vi "Main.vi"(8 "error in":errorcluster, 11 "Message Log in":refnum<class "Message Log.lvclass">) -> (0 "error out":errorcluster, 3 "Message Log out":refnum<class "Message Log.lvclass">)   [LabVIEW 2017, in "Message Log.lvclass"]
doc: "The <b>Queued Message Handler</b> of the Worker that owns this VI."
uses:
  Message Log.lvclass
  C:/Program Files (x86)/National Instruments/LabVIEW 2017/vi.lib/addons/_Workers/Library/Classes/Worker/Worker.lvclass
  Message Log Columns.ctl
  Buttons/Sort Button.ctl
  Buttons/Logging Button.ctl
  Buttons/Clear Filter Button.ctl
  Buttons/Undo Filter Button.ctl
  Buttons/Filter Button.ctl
  Buttons/Resize Button.ctl
  Buttons/Pause Button.ctl
  Buttons/WID Button.ctl
  Buttons/Open Application Manager.ctl
  <vilib>/Utility/miscctls.llb/LVRowAndColumnUnsignedTypeDef.ctl
  FP Refs.ctl
  Message Log.lvclass/Message Log.ctl
  <vilib>/addons/_Workers/Library/Classes/Worker/Worker.lvclass/Worker.ctl
  rql_Update Message Log Columns.ctl
  rql_EHL Logging - Value Change.ctl
  rql_EHL Pause - Value Change.ctl
  rql_EHL WID - Value Change.ctl
  Initialization Data.ctl
  Response Cases.ctl
  <vilib>/addons/_Workers/Library/Case Label.ctl
  Common VIs/Message Log ID.ctl
  Config Data.ctl
  <vilib>/Utility/miscctls.llb/LVRectTypeDef.ctl
  <vilib>/addons/_Workers/Library/Classes/Message/Priority.ctl
  rsp_Message Log Shutdown.ctl
  rsp_Message Log Exited.ctl
  Message Log Filter Data.ctl
  String Filter Type.ctl
  rql_EHL Message Log - Mouse Down.ctl
  Listbox Selection.ctl
  <vilib>/Utility/miscctls.llb/LVRowAndColumnTypeDef.ctl
  rql_EHL Sort - Value Change.ctl
  rql_EHL Resize - Value Change.ctl
  rql_EHL Undo Filter - Value Change.ctl
  rqp_Show Front Panel.ctl
  rwr_Get Shutdown Data Reply.ctl
  rqp_Filter as Enque Worker.ctl
  rqp_Filter as Deque Worker.ctl
  Format Message Log Data.vi
  Log Message to File.vi
  Replace ID with Alias.vi
  <vilib>/Platform/browser.llb/Open URL in Default Browser (string).vi
  <vilib>/addons/_Workers/Library/Classes/Worker/Worker.lvclass
  <vilib>/addons/_Workers/Library/Workers.lvlib
  <vilib>/addons/_Workers/Library/Classes/Message Queue/Message Queue.lvclass
  <vilib>/addons/_Workers/Library/Classes/Message/Message.lvclass
panel:
  in  "Show App Mgr":T1
  out "Warning : Message Backlog":i32
  out "Visible ML Columns":bool[](array[boolean])
  out "Title":string="Worker A  (127.0.0.1)"
  in  "WID":T2
  in  "Pause":T3
  in  "Resize":T4
  in  "Filter":T5
  in  "Undo":T6
  in  "Clear":T7
  in  "Logging":T8
  in  "Filter String":string caption="String to Filter"
  in  "Sort":T9
  in  "Column":T10
  in  "Filter Type":enum16{"string only", "match pattern"}(ring)
  in  "Filter Log":i32(listbox)=-1
  in  "Message Log":i32(listbox)=-1
  out "Message Box":string
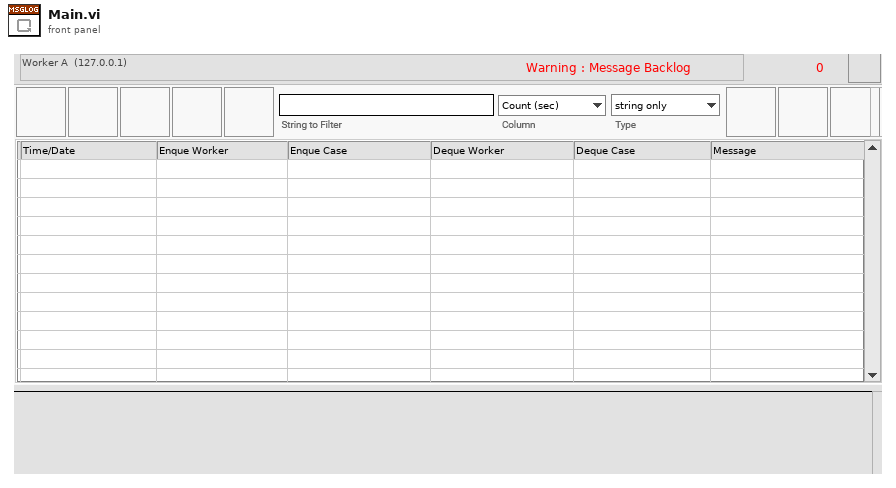
[diagram p1: front panel]
types:
  T1 = typedef "Open Application Manager.ctl" = bool
  T2 = typedef "WID Button.ctl" = bool
  T3 = typedef "Pause Button.ctl" = bool
  T4 = typedef "Resize Button.ctl" = bool
  T5 = typedef "Filter Button.ctl" = bool
  T6 = typedef "Undo Filter Button.ctl" = bool
  T7 = typedef "Clear Filter Button.ctl" = bool
  T8 = typedef "Logging Button.ctl" = bool
  T9 = typedef "Sort Button.ctl" = bool
  T10 = typedef "Message Log.lvclass/Message Log Columns.ctl" = enum16{"Count (sec)", "Time/Date", "Enque Worker", "Enque Case", "Deque Worker", "Deque Case", "Priority", "Message"}
  T11 = typedef "Message Log.lvclass/FP Refs.ctl" = cluster{"Message Log.Ref":refnum<vi>, "VisibleMLColumns.Ref":refnum<vi>, "Filter Type.Ref":refnum<vi>, "Column.Ref":refnum<vi>, "Filter String.Ref":refnum<vi>, "Filter Log.Ref":refnum<vi>, "MessageBox.Ref":refnum<vi>, "MessageBacklog.Ref":refnum<vi>, "Title.Ref":refnum<vi>}
  T12 = typedef "LVRowAndColumnUnsignedTypeDef.ctl" = cluster{"Row":u32, "Column":u32}
  T13 = typedef "LVPointTypeDef.ctl" = cluster{"Horizontal":i16, "Vertical":i16}
  T14 = typedef "Message Log.lvclass/Initialization Data.ctl" = cluster{"Response Cases":T15, "Message Log ID":T17, "Config Data":T18}
  T15 = typedef "Message Log.lvclass/Response Cases.ctl" = cluster{"Message Log Exited":T16, "Go to MHL Case":T16, "Open Running VI":T16, "Message Log Shutdown Data":T16, "Show Application Manager":T16}
  T16 = typedef "Workers.lvlib/Case Label.ctl" = string
  T17 = typedef "Message Log ID.ctl" = cluster{"Head Worker ID":string, "IP Address":string}
  T18 = typedef "Message Log.lvclass/Config Data.ctl" = cluster{"Max Num Rows":i32, "Visible Columns":bool[], "Splitter Position":i32, "Column Widths":u32[], "WinBounds":T19, "FP.State":enum32{"Invalid", "Standard", "Closed", "Hidden", "Minimized", "Maximized"}, "Monitor":u16, "Logging":bool, "LogBaseFolder":path}
  T19 = typedef "LVRectTypeDef.ctl" = cluster{"Left":i16, "Top":i16, "Right":i16, "Bottom":i16}
  T20 = typedef "Workers.lvlib/Message.lvclass/Priority.ctl" = enum16{"Low", "Normal", "High"}
  T21 = typedef "Message Log.lvclass/rql_Update Message Log Columns.ctl" = cluster{"Boolean":bool}
  T22 = typedef "Message Log.lvclass/rsp_Message Log Shutdown.ctl" = cluster{"Config Data":T18}
  T23 = typedef "Message Log.lvclass/rsp_Message Log Exited.ctl" = cluster{"Message Log ID":T17}
  T24 = typedef "Message Log.lvclass/Message Log Filter Data.ctl" = cluster{"Element":string, "Column":T10, "Filter Type":T25}
  T25 = typedef "Message Log.lvclass/String Filter Type.ctl" = enum16{"string only", "match pattern"}
  T26 = typedef "Message Log.lvclass/rql_EHL Message Log - Mouse Down.ctl" = cluster{"Listbox Selection":T27}
  T27 = typedef "Message Log.lvclass/Listbox Selection.ctl" = cluster{"Cell Position":T28, "Row":string[]}
  T28 = typedef "LVRowAndColumnTypeDef.ctl" = cluster{"Row":i32, "Column":i32}
  T29 = typedef "Message Log.lvclass/rql_EHL Pause - Value Change.ctl" = cluster{"Boolean":bool}
  T30 = typedef "Message Log.lvclass/rql_EHL WID - Value Change.ctl" = cluster{"Boolean":bool}
  T31 = typedef "Message Log.lvclass/rql_EHL Sort - Value Change.ctl" = cluster{"String":string}
  T32 = typedef "Message Log.lvclass/rql_EHL Resize - Value Change.ctl" = cluster{"String":string}
  T33 = typedef "Message Log.lvclass/rql_EHL Undo Filter - Value Change.ctl" = cluster{"String":string}
  T34 = typedef "Message Log.lvclass/rql_EHL Logging - Value Change.ctl" = cluster{"Boolean":bool}
  T35 = typedef "Message Log.lvclass/rqp_Show Front Panel.ctl" = cluster{"String":string}
  T36 = typedef "Message Log.lvclass/rwr_Get Shutdown Data Reply.ctl" = cluster{"Config Data":T18}
  T37 = typedef "Message Log.lvclass/rqp_Filter as Enque Worker.ctl" = cluster{"Worker ID":string}
  T38 = typedef "Message Log.lvclass/rqp_Filter as Deque Worker.ctl" = cluster{"Worker ID":string}
  T39 = typedef "LVPoint32TypeDef.ctl" = cluster{"Horizontal":i32, "Vertical":i32}
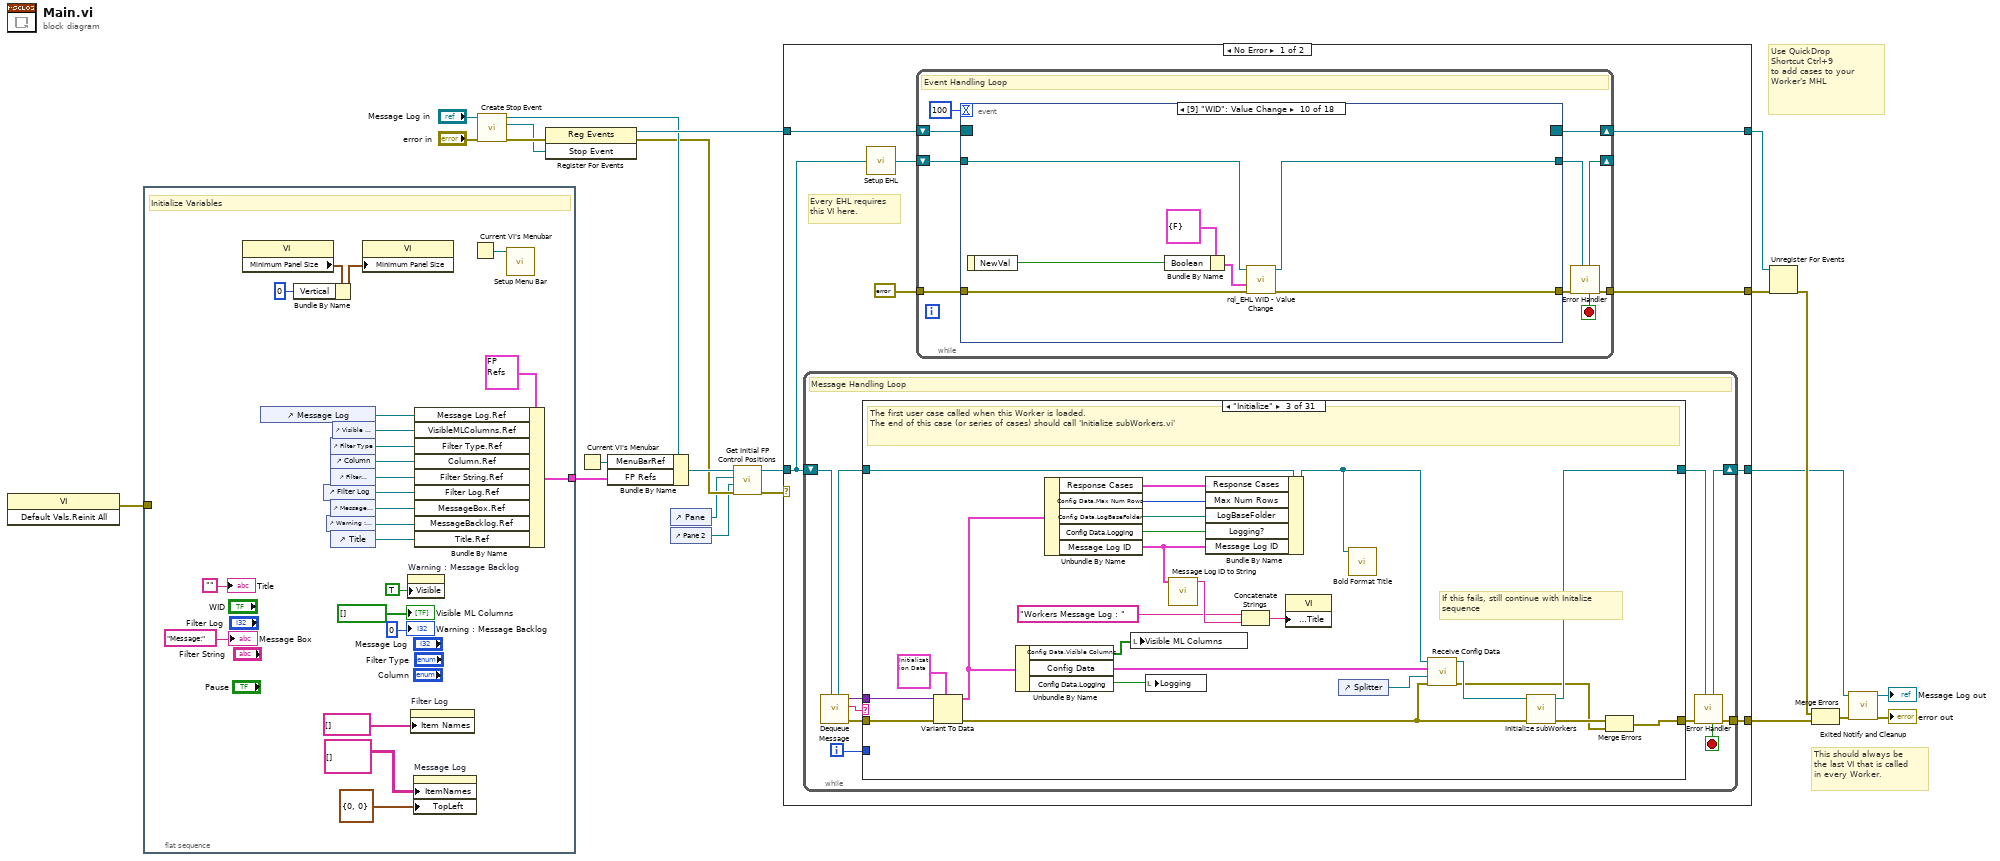
[diagram p0: block diagram]
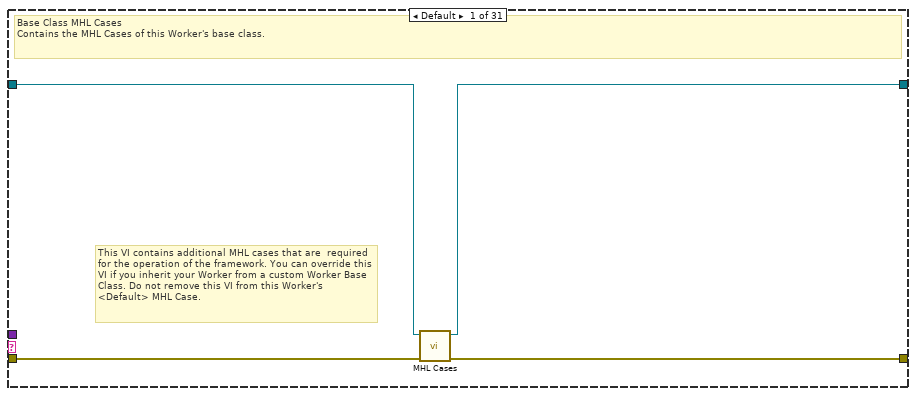
[diagram p2: hidden frame]
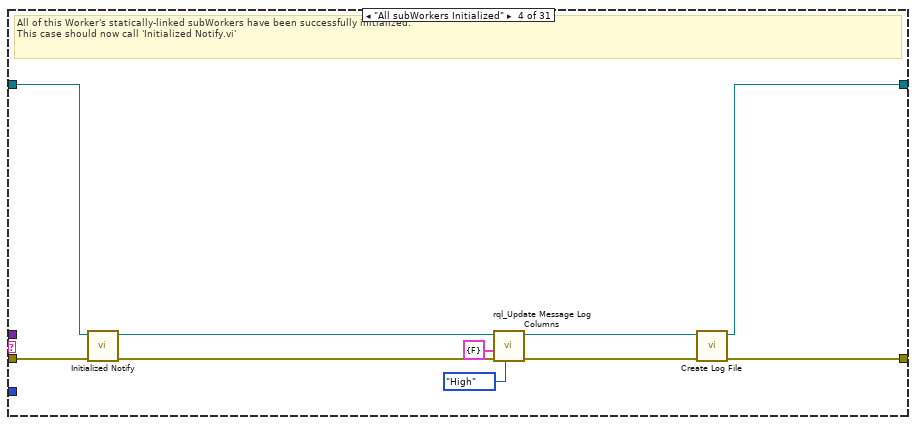
[diagram p4: hidden frame]
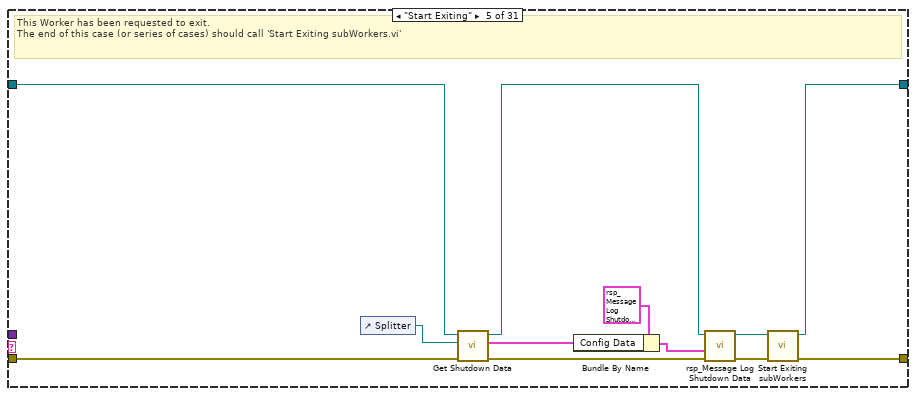
[diagram p5: hidden frame]
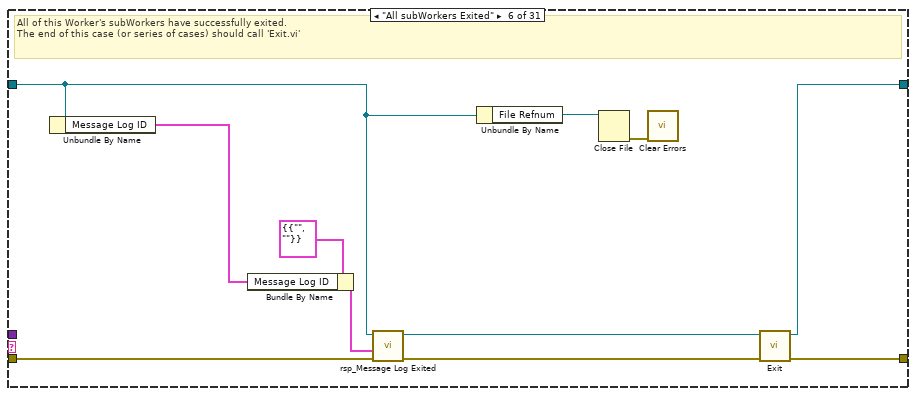
[diagram p6: hidden frame]
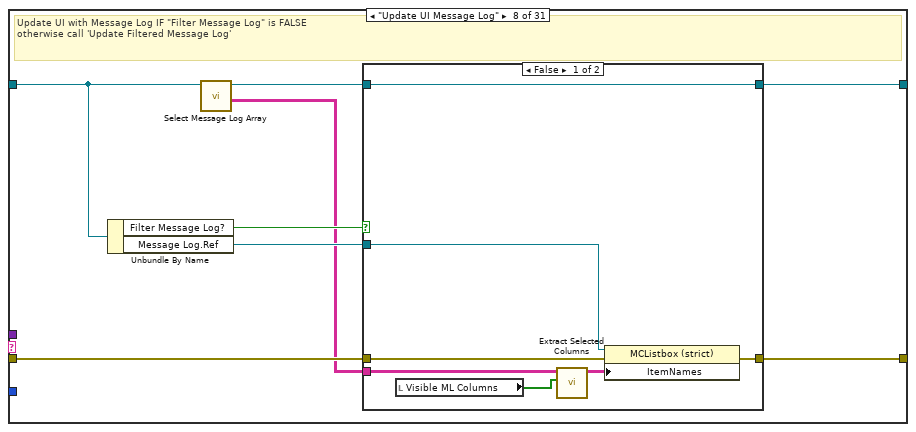
[diagram p8: hidden frame]
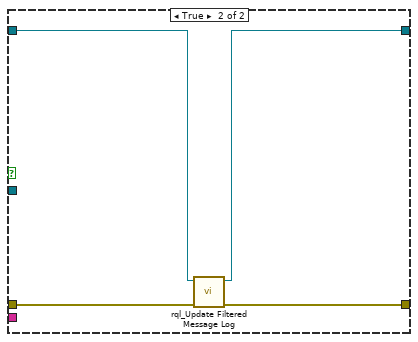
[diagram p9: hidden frame]
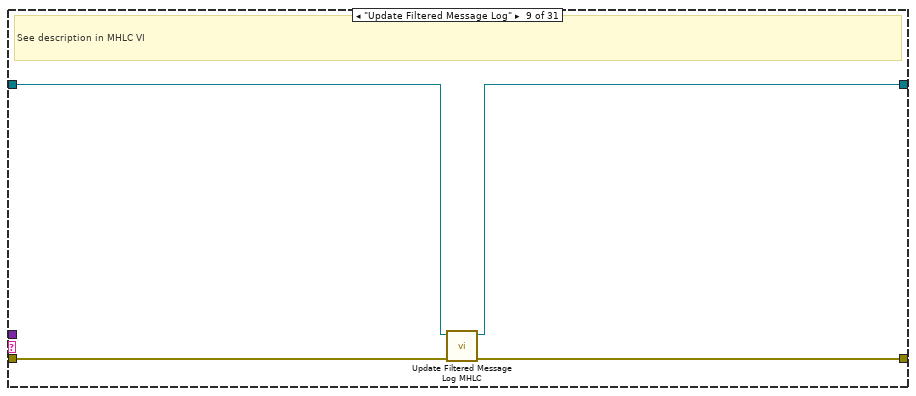
[diagram p10: hidden frame]
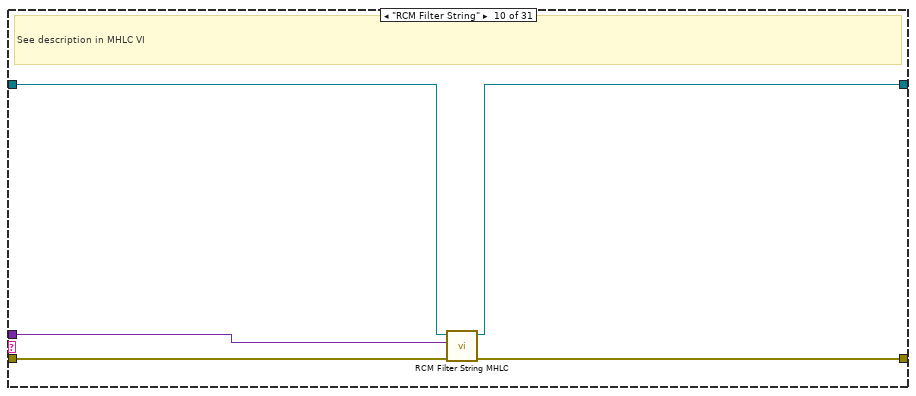
[diagram p11: hidden frame]
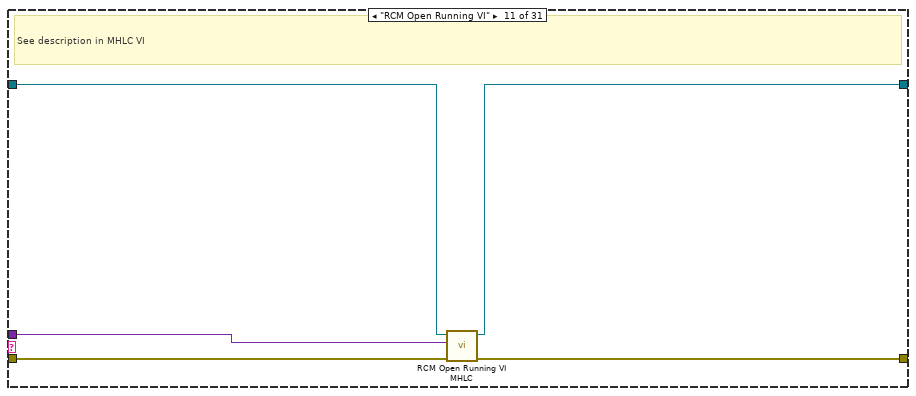
[diagram p12: hidden frame]
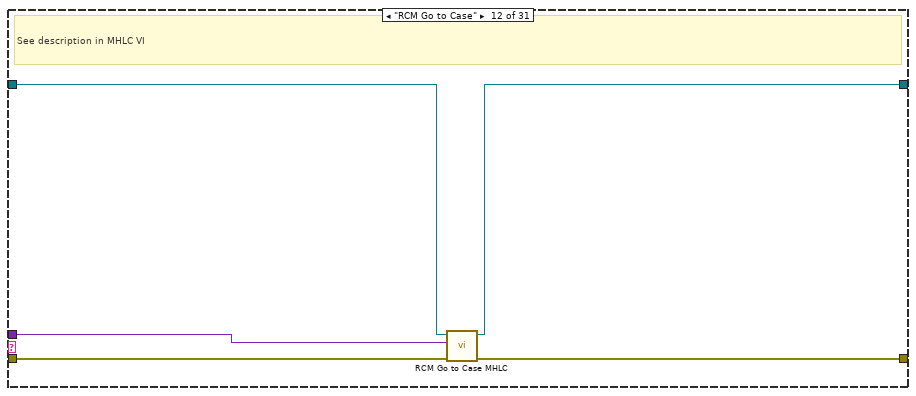
[diagram p13: hidden frame]
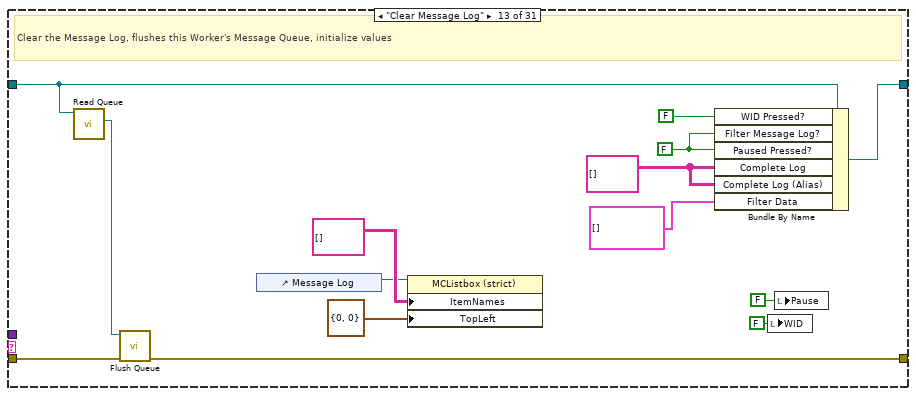
[diagram p14: hidden frame]
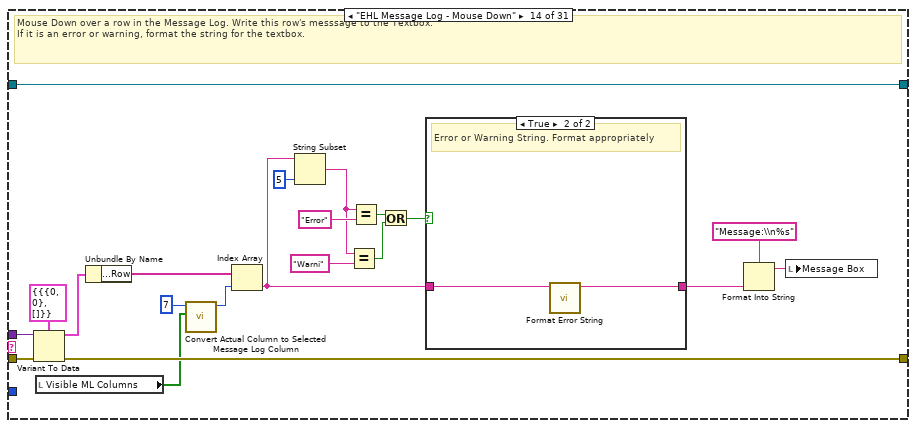
[diagram p15: hidden frame]
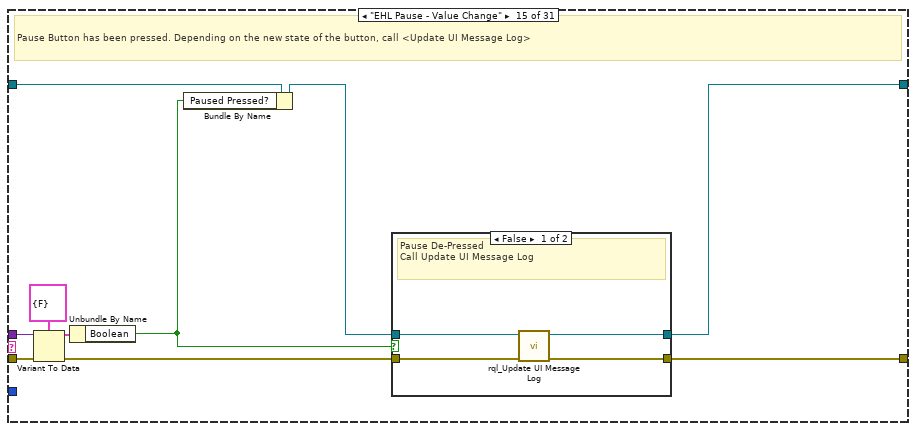
[diagram p17: hidden frame]
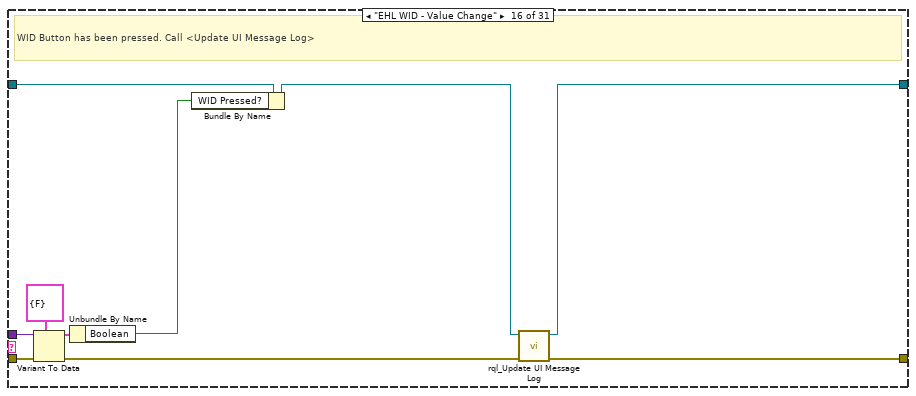
[diagram p19: hidden frame]
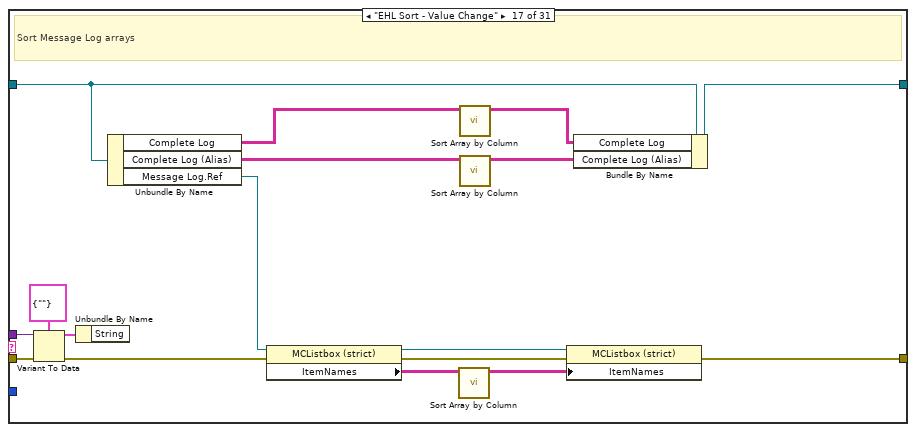
[diagram p20: hidden frame]
diagram:
  # "Use QuickDrop\nShortcut Ctrl+9\nto add cases to your\nWorker's MHL"
  # "This should always be the last VI that is called in every Worker."
  n1 = invoke class="VI" method="Default Vals.Reinit All"() -> (error out=w10:errorcluster)  [unwired: 3 in, 2 out]
  n2 = flat-sequence {
    tunnel: w10 -> [_]
    tunnel: [w45] -> w8
    frame #0 {
      # "Initialize Variables"
      n3 = property class="VI"() -> ("Minimum Panel Size"=w32:T13)  [unwired: 2 in, 2 out]
      n4 = control-ref of="Message Log"() -> (w44:refnum<vi>)
      n5 = Bundle By Name(cluster=w32, "Vertical"=i16 0) -> (w31:T13)
      n6 = control-ref of="Filter Log"() -> (w40:refnum<vi>)
      n7 = control-ref of="Warning : Message Backlog"() -> (w38:refnum<vi>)
      n8 = control-ref of="Filter Type"() -> (w42:refnum<vi>)
      n9 = control-ref of="Column"() -> (w26:refnum<vi>)
      n10 = control-ref of="Filter String"() -> (w41:refnum<vi>)
      n11 = control-ref of="Message Box"() -> (w39:refnum<vi>)
      n12 = control-ref of="Title"() -> (w25:refnum<vi>)
      n13 = control-ref of="Visible ML Columns"() -> (w43:refnum<vi>)
      n14 = property class="VI"("Minimum Panel Size"=w31) -> ()  [unwired: 2 in, 2 out]
      n15 = property on="Warning : Message Backlog" class="DigNum (strict)"("Visible"=TRUE) -> ()  [unwired: 2 in, 2 out]
      n16 = property on="Filter Log" class="LstBox (strict)"("Item Names"=string[] [] ("Sorted Array Out")) -> ()  [unwired: 2 in, 2 out]
      n17 = property on="Message Log" class="MCListbox (strict)"("ItemNames"=string[][] [] ("Sorted Array Out"), "TopLeft"=T12 {"Row"=0, "Column"=0} ("Top Left Visible Cell")) -> ()  [unwired: 2 in, 2 out]
      n18 = Bundle By Name(cluster=T11 {"Message Log.Ref"=refnum, "VisibleMLColumns.Ref"=refnum, "Filter Type.Ref"=refnum, "Column.Ref"=refnum, "Filter String.Ref"=refnum, "Filter Log.Ref"=refnum, "MessageBox.Ref"=refnum, "MessageBacklog.Ref"=refnum, "Title.Ref"=refnum} ("Data"), "Message Log.Ref"=w44, "VisibleMLColumns.Ref"=w43, "Filter Type.Ref"=w42, "Column.Ref"=w26, "Filter String.Ref"=w41, "Filter Log.Ref"=w40, "MessageBox.Ref"=w39, "MessageBacklog.Ref"=w38, "Title.Ref"=w25) -> (w45:T11)
      n19 = Current VI's Menubar() -> (w29:refnum<k9>)
      n20 = call "Setup Menu Bar.vi"("menu reference"=w29) -> ()  [unwired: 10 in, 1 out]
      "Message Box" <- "Message:" ("TextBox")
      "Warning : Message Backlog" <- 0 ("Warning : Message Backlog")
      "Visible ML Columns" <- bool[] [] ("Visible ML Columns")
      "Title" <- ""
    }
  }
  n21 = call-dynamic "Create Stop Event.vi"("error in"="error in", "Worker"="Message Log in") -> ("error out"=w18:errorcluster, "Stop Event"=w15:refnum<user-event>, "Worker out"=w9:refnum<class "Message Log.lvclass">)  [unwired: 7 in]
  n22 = register-events(error in=w18, w15) -> (reference out=w17:refnum<event-registration>, error out=w6:errorcluster)  [unwired: 1 in]
  n23 = Current VI's Menubar() -> (w3:refnum<k9>)
  n24 = Bundle By Name(cluster=w9, "MenuBarRef"=w3, "FP Refs"=w8) -> (w7:refnum<class "Message Log.lvclass">)
  n25 = control-ref of="Pane"() -> (w5:refnum<vi>)
  n26 = control-ref of="Pane"() -> ()  [unwired: 1 out]
  n27 = control-ref of="Pane 2"() -> (w4:refnum<vi>)
  n28 = call "Get Initial FP Control Positions.vi"("error in (no error)"=w6, "Pane 2"=w4, "Pane"=w5, "Message Log in"=w7) -> ("error out"=w2:errorcluster, "Message Log out"=w1:refnum<class "Message Log.lvclass">)  [unwired: 6 in]
  n29 = case shown="No Error" w2 {
    tunnel: w1 -> [w49 w539]
    tunnel: [w47 w540] -> w16
    tunnel: w17 -> [w54 w541]
    tunnel: [w51 w542] -> w22
    tunnel: [w53 w541] -> w21
    tunnel: [w48 w538] -> w19
    selector: w2 -> [_ w542]
    frame No Error {
      # "Every EHL requires\nthis VI here."
      n30 = while {
        shift-right: [w63] -> w48
        shift-left: w49 -> [w65]
        tunnel: [w64] -> w47
        i -> [w56]
        stop <- w57 stop-if-true
        # "Message Handling Loop"
        n31 = call-dynamic "Dequeue Message.vi"("Worker"=w65) -> ("error out"=w62:errorcluster, "Case out"=w58:string, "Data out"=w55:variant, "Worker out"=w60:refnum<class "Message Log.lvclass">)  [unwired: 6 in, 1 out]
        n32 = case "Worker MHL Case Structure (DO NOT CHANGE LABEL NAME)" shown="\"Initialize\"" w58 {
          tunnel: w62 -> [w69 w70 w93 w104 w111 w128 w130 w138 w153 w158 w163 w168 w172 w203 w216 w232 w249 w257 w261 w269 w280 w284 w300 w326 w328 w334 w341 w361 w378 w380 w386]
          tunnel: [w68 w70 w82 w98 w117 w127 w130 w136 w151 w157 w162 w167 w171 w201 w211 w227 w238 w250 w260 w264 w270 w283 w288 w319 w328 w332 w340 w356 w373 w380 w384] -> w61
          tunnel: w60 -> [w67 w71 w91 w105 w107 w119 w129 w137 w150 w156 w161 w166 w170 w202 w210 w226 w240 w253 w259 w263 w278 w282 w289 w325 w327 w333 w336 w354 w371 w379 w388]
          tunnel: [w66 w71 w94 w96 w116 w126 w129 w134 w152 w155 w160 w165 w176 w202 w209 w225 w237 w253 w258 w262 w274 w281 w286 w317 w327 w333 w339 w355 w372 w379 w383] -> w59
          tunnel: w56 -> [_ _ _ _ _ _ _ _ _ _ _ _ _ _ _ _ _ _ _ _ _ _ _ _ _ _ _ _ _ _ _]
          tunnel: w55 -> [_ _ w92 _ _ _ _ _ _ w154 w159 w164 _ w199 w213 w229 w247 w255 _ w266 _ _ w297 w322 _ w330 _ w358 w375 _ w387]
          frame Default {
            # "This VI contains additional MHL cases that are  required for the operation of the framework. You can override this VI if you inherit your Worker from a custom Worker Base Class. Do not remove this VI from this Worker's <Default> MHL Case."
            # "Base Class MHL Cases\nContains the MHL Cases of this Worker's base class."
            n33 = call-dynamic "MHL Cases.vi"("error in"=w69, "Worker in"=w67) -> ("error out"=w68:errorcluster, "Worker out"=w66:refnum<class "Message Log.lvclass">)  [unwired: 8 in]
          }
          frame "------------ FRAMEWORK CASES -----------" {
            # "Start of Workers Framework Cases"
          }
          frame "Initialize" {
            # "If this fails, still continue with Initalize\nsequence"
            # "The first user case called when this Worker is loaded.\nThe end of this case (or series of cases) should call 'Initialize subWorkers.vi'"
            n34 = Variant To Data(error in=w93, type=T14 {"Response Cases"={"Message Log Exited"="", "Go to MHL Case"="", "Open Running VI"="", "Message Log Shutdown Data"="", "Show Application Manager"=""}, "Message Log ID"={"Head Worker ID"="", "IP Address"=""}, "Config Data"={"Max Num Rows"=0, "Visible Columns"=[], "Splitter Position"=0, "Column Widths"=[], "WinBounds"={"Left"=0, "Top"=0, "Right"=0, "Bottom"=0}, "FP.State"=enum."Invalid", "Monitor"=0, "Logging"=FALSE, "LogBaseFolder"=path ""}} ("Initialization Data"), Variant=w92) -> (data=w79:T14, error out=w81:errorcluster)
            n35 = Unbundle By Name(w79) -> ("Config Data.Visible Columns"=w76:bool[], "Config Data"=w78:T18, "Config Data.Logging"=w75:bool)
            n36 = Unbundle By Name(w79) -> ("Response Cases"=w89:T15, "Config Data.Max Num Rows"=w87:i32, "Config Data.LogBaseFolder"=w74:path, "Config Data.Logging"=w73:bool, "Message Log ID"=w88:T17)
            n37 = local write "Visible ML Columns"(w76) -> ()
            n38 = local write "Logging"(w75) -> ()
            n39 = call "Message Log ID to String.vi"("Message Log ID"=w88) -> ("Message Log ID String"=w86:string)  [unwired: 10 in]
            n40 = Bundle By Name(cluster=w91, "Response Cases"=w89, "Max Num Rows"=w87, "LogBaseFolder"=w74, "Logging?"=w73, "Message Log ID"=w88) -> (w72:refnum<class "Message Log.lvclass">)
            n41 = Concatenate Strings("Workers Message Log : " ("string"), w86) -> (w85:string)
            n42 = property class="VI"("Front Panel.Title"=w85) -> ()  [unwired: 2 in, 2 out]
            n43 = control-ref of="Splitter"() -> (w77:refnum<vi>)
            n44 = call "Bold Format Title.vi"("Message Log in"=w72) -> ()  [unwired: 11 in]
            n45 = call "Receive Config Data.vi"("error in (no error)"=w81, "Splitter"=w77, "Config Data"=w78, "Message Log in"=w72) -> ("error out"=w80:errorcluster, "Message Log out"=w83:refnum<class "Message Log.lvclass">)  [unwired: 6 in]
            n46 = call-dynamic "Initialize subWorkers.vi"("error in"=w81, "Worker"=w83) -> ("error out"=w95:errorcluster, "dup Worker out"=w94:refnum<class "Message Log.lvclass">)  [unwired: 8 in]
            n47 = Merge Errors(w95, w80) -> (w82:errorcluster)
          }
          frame "All subWorkers Initialized" {
            # "All of this Worker's statically-linked subWorkers have been successfully initialized.\nThis case should now call 'Initialized Notify.vi'"
            n48 = call-dynamic "Initialized Notify.vi"("error in"=w104, "Worker"=w105) -> ("error out"=w103:errorcluster, "dup Worker out"=w101:refnum<class "Message Log.lvclass">)  [unwired: 8 in]
            n49 = call "rql_Update Message Log Columns.vi"("Message Priority"=Priority."High", "error in"=w103, "Data in"=T21 {"Boolean"=FALSE}, "Message Log in"=w101) -> ("error out"=w102:errorcluster, "dup Message Log out"=w97:refnum<class "Message Log.lvclass">)  [unwired: 6 in]
            n50 = call "Create Log File.vi"("error in (no error)"=w102, "Message Log in"=w97) -> ("error out"=w98:errorcluster, "Message Log out"=w96:refnum<class "Message Log.lvclass">)  [unwired: 8 in]
          }
          frame "Start Exiting" {
            # "This Worker has been requested to exit. \nThe end of this case (or series of cases) should call 'Start Exiting subWorkers.vi'"
            n51 = control-ref of="Splitter"() -> (w113:refnum<vi>)
            n52 = call "Get Shutdown Data.vi"("error in (no error)"=w111, "Splitter"=w113, "Message Log in"=w107) -> ("error out"=w112:errorcluster, "Data"=w108:T18, "Message Log out"=w106:refnum<class "Message Log.lvclass">)  [unwired: 6 in]
            n53 = Bundle By Name(cluster=T22 {"Config Data"={"Max Num Rows"=0, "Visible Columns"=[], "Splitter Position"=0, "Column Widths"=[], "WinBounds"={"Left"=0, "Top"=0, "Right"=0, "Bottom"=0}, "FP.State"=enum."Invalid", "Monitor"=0, "Logging"=FALSE, "LogBaseFolder"=path ""}} ("Data in"), "Config Data"=w108) -> (w109:T22)
            n54 = call "rsp_Message Log Shutdown Data.vi"("error in"=w112, "Data in"=w109, "Message Log in"=w106) -> ("error out"=w115:errorcluster, "dup Message Log out"=w114:refnum<class "Message Log.lvclass">)  [unwired: 7 in]
            n55 = call-dynamic "Start Exiting subWorkers.vi"("error_in"=w115, "Worker"=w114) -> ("error out"=w117:errorcluster, "dup Worker out"=w116:refnum<class "Message Log.lvclass">)  [unwired: 8 in]
          }
          frame "All subWorkers Exited" {
            # "All of this Worker's subWorkers have successfully exited. \nThe end of this case (or series of cases) should call 'Exit.vi'"
            n56 = Unbundle By Name(w119) -> ("Message Log ID"=w121:T17)
            n57 = Bundle By Name(cluster=T23 {"Message Log ID"={"Head Worker ID"="", "IP Address"=""}} ("Data in"), "Message Log ID"=w121) -> (w122:T23)
            n58 = call "rsp_Message Log Exited.vi"("error in"=w128, "Data in"=w122, "Message Log in"=w119) -> ("error out"=w125:errorcluster, "dup Message Log out"=w124:refnum<class "Message Log.lvclass">)  [unwired: 7 in]
            n59 = Unbundle By Name(w119) -> ("File Refnum"=w120:refnum<file>)
            n60 = Close File(refnum=w120) -> (error out=w118:errorcluster)  [unwired: 1 in, 1 out]
            n61 = call <vilib>:"Clear Errors.vi"("error in (no error)"=w118) -> ()  [unwired: 5 in, 2 out]
            n62 = call-dynamic "Exit.vi"("error_in"=w125, "Worker"=w124) -> ("error out"=w127:errorcluster, "dup Worker out"=w126:refnum<class "Message Log.lvclass">)  [unwired: 8 in]
          }
          frame "------------- LOCAL API CASES -------------" {
            # "Start of Workers Local API Cases"
          }
          frame "Update UI Message Log" {
            # "Update UI with Message Log IF \"Filter Message Log\" is FALSE\notherwise call 'Update Filtered Message Log'"
            n63 = Unbundle By Name(w137) -> ("Filter Message Log?"=w133:bool, "Message Log.Ref"=w132:refnum<vi>)
            n64 = call "Select Message Log Array.vi"("Message Log in"=w137) -> ("Selected Array"=w131:string[][], "Message Log out"=w135:refnum<class "Message Log.lvclass">)  [unwired: 9 in]
            n65 = case shown="False" w133 {
              tunnel: w138 -> [w143 w149]
              tunnel: [w142 w148] -> w136
              tunnel: w135 -> [w145 w147]
              tunnel: [w145 w146] -> w134
              tunnel: w132 -> [w144 _]
              tunnel: w131 -> [w140 _]
              frame False {
                n66 = local read "Visible ML Columns"() -> (w139:bool[])
                n67 = call "Extract Selected Columns.vi"("Visible ML Columns"=w139, "Array in"=w140) -> ("Selected Columns out"=w141:string[][])  [unwired: 9 in]
                n68 = property class="MCListbox (strict)"(reference=w144, error in=w143, "ItemNames"=w141) -> (error out=w142:errorcluster)  [unwired: 1 out]
              }
              frame True {
                n69 = call "rql_Update Filtered Message Log.vi"("error in"=w149, "Message Log in"=w147) -> ("error out"=w148:errorcluster, "dup Message Log out"=w146:refnum<class "Message Log.lvclass">)  [unwired: 8 in]
              }
            }
          }
          frame "Update Filtered Message Log" {
            # "See description in MHLC VI"
            n70 = call "Update Filtered Message Log MHLC.vi"("error in (no error)"=w153, "Message Log in"=w150) -> ("error out"=w151:errorcluster, "Message Log out"=w152:refnum<class "Message Log.lvclass">)  [unwired: 8 in]
          }
          frame "RCM Filter String" {
            # "See description in MHLC VI"
            n71 = call "RCM Filter String MHLC.vi"("error in (no error)"=w158, "Data"=w154, "Message Log in"=w156) -> ("error out"=w157:errorcluster, "Message Log out"=w155:refnum<class "Message Log.lvclass">)  [unwired: 7 in]
          }
          frame "RCM Open Running VI" {
            # "See description in MHLC VI"
            n72 = call "RCM Open Running VI MHLC.vi"("error in (no error)"=w163, "Data"=w159, "Message Log in"=w161) -> ("error out"=w162:errorcluster, "Message Log out"=w160:refnum<class "Message Log.lvclass">)  [unwired: 7 in]
          }
          frame "RCM Go to Case" {
            # "See description in MHLC VI"
            n73 = call "RCM Go to Case MHLC.vi"("error in (no error)"=w168, "Data"=w164, "Message Log in"=w166) -> ("error out"=w167:errorcluster, "Message Log out"=w165:refnum<class "Message Log.lvclass">)  [unwired: 7 in]
          }
          frame "Clear Message Log" {
            w179 = FALSE ("Update Message Log?")
            w181 = string[][] [] ("Sorted Array Out")
            # "Clear the Message Log, flushes this Worker's Message Queue, initialize values"
            n74 = call <vilib>:"Read Queue.vi"("Worker_"=w170) -> ("Message Queue out"=w169:refnum<class "Message Queue.lvclass">)  [unwired: 9 in, 1 out]
            n75 = call <vilib>:"Flush Queue.vi"("error in (no error)"=w172, "Message Queue"=w169) -> ("error out"=w171:errorcluster)  [unwired: 7 in, 2 out]
            n76 = control-ref of="Message Log"() -> (w173:refnum<vi>)
            n77 = property class="MCListbox (strict)"(reference=w173, "ItemNames"=string[][] [] ("Sorted Array Out"), "TopLeft"=T12 {"Row"=0, "Column"=0} ("Top Left Visible Cell")) -> ()  [unwired: 1 in, 2 out]
            n78 = Bundle By Name(cluster=w170, "WID Pressed?"=FALSE ("Full ID Pressed?"), "Filter Message Log?"=w179, "Paused Pressed?"=w179, "Complete Log"=w181, "Complete Log (Alias)"=w181, "Filter Data"=T24[] []) -> (w176:refnum<class "Message Log.lvclass">)
            n79 = local write "WID"(T2 FALSE ("ID")) -> ()
            n80 = local write "Pause"(T3 FALSE ("Pause")) -> ()
          }
          frame "EHL Message Log - Mouse Down" {
            # "Mouse Down over a row in the Message Log. Write this row's messsage to the Textbox.\nIf it is an error or warning, format the string for the textbox."
            n81 = Variant To Data(error in=w203, type=T26 {"Listbox Selection"={"Cell Position"={"Row"=0, "Column"=0}, "Row"=[]}} ("Data"), Variant=w199) -> (data=w198:T26, error out=w201:errorcluster)
            n82 = local read "Visible ML Columns"() -> (w196:bool[])
            n83 = Unbundle By Name(w198) -> ("Listbox Selection.Row"=w195:string[])
            n84 = call "Convert Actual Column to Selected Message Log Column.vi"("Visible ML Columns"=w196, "Actual Column"=7) -> ("Selected Column"=w194:i32)  [unwired: 9 in]
            n85 = Index Array(array=w195, index=w194) -> (element=w186:string)
            n86 = String Subset(string=w186, length (rest)=5 ("length (rest)")) -> (substring=w189:string)  [unwired: 1 in]
            n87 = Equal?(x=w189, y="Warni") -> (x = y?=w188:bool)
            n88 = Equal?(x=w189, y="Error") -> (x = y?=w191:bool)
            n89 = Or(x=w191, y=w188) -> (x .or. y?=w187:bool)
            n90 = case shown="True" w187 {
              tunnel: w186 -> [w204 w206]
              tunnel: [w204 w205] -> w184
              frame False {
                # "Not Error or Warning. Pass message string through directly"
              }
              frame True {
                # "Error or Warning String. Format appropriately"
                n91 = call "Format Error String.vi"("raw error string"=w206) -> ("formatted error string"=w205:string)  [unwired: 10 in]
              }
            }
            n92 = Format Into String(format string="Message:\\n%s", w184) -> (resulting string=w183:string)  [unwired: 2 in, 1 out]
            n93 = local write "Message Box"(w183) -> ()
          }
          frame "EHL Pause - Value Change" {
            # "Pause Button has been pressed. Depending on the new state of the button, call <Update UI Message Log>"
            n94 = Variant To Data(error in=w216, type=T29 {"Boolean"=FALSE} ("Data"), Variant=w213) -> (data=w212:T29, error out=w215:errorcluster)
            n95 = Unbundle By Name(w212) -> ("Boolean"=w207:bool)
            n96 = Bundle By Name(cluster=w210, "Paused Pressed?"=w207) -> (w208:refnum<class "Message Log.lvclass">)
            n97 = case shown="False" w207 {
              tunnel: w215 -> [w220 w221]
              tunnel: [w219 w221] -> w211
              tunnel: [w218 w222] -> w209
              tunnel: w208 -> [w217 w222]
              frame False {
                # "Pause De-Pressed\nCall Update UI Message Log"
                n98 = call "rql_Update UI Message Log.vi"("error in"=w220, "Message Log in"=w217) -> ("error out"=w219:errorcluster, "dup Message Log out"=w218:refnum<class "Message Log.lvclass">)  [unwired: 8 in]
              }
              frame True {
                # "Paused pressed. Nothing to do."
              }
            }
          }
          frame "EHL WID - Value Change" {
            # "WID Button has been pressed. Call <Update UI Message Log>"
            n99 = Variant To Data(error in=w232, type=T30 {"Boolean"=FALSE} ("Data"), Variant=w229) -> (data=w228:T30, error out=w231:errorcluster)
            n100 = Unbundle By Name(w228) -> ("Boolean"=w223:bool)
            n101 = Bundle By Name(cluster=w226, "WID Pressed?"=w223) -> (w224:refnum<class "Message Log.lvclass">)
            n102 = call "rql_Update UI Message Log.vi"("error in"=w231, "Message Log in"=w224) -> ("error out"=w227:errorcluster, "dup Message Log out"=w225:refnum<class "Message Log.lvclass">)  [unwired: 8 in]
          }
          frame "EHL Sort - Value Change" {
            # "Sort Message Log arrays"
            n103 = Variant To Data(error in=w249, type=T31 {"String"=""} ("Data"), Variant=w247) -> (data=w246:T31, error out=w239:errorcluster)
            n104 = Unbundle By Name(w246) -> ()  [unwired: 1 out]
            n105 = Unbundle By Name(w240) -> ("Complete Log"=w235:string[][], "Complete Log (Alias)"=w234:string[][], "Message Log.Ref"=w241:refnum<vi>)
            n106 = property class="MCListbox (strict)"(reference=w241, error in=w239) -> (reference out=w245:refnum<vi>, error out=w242:errorcluster, "ItemNames"=w243:string[][])
            n107 = call "Sort Array by Column.vi"("Unsorted Array"=w243) -> ("Sorted Array"=w244:string[][])  [unwired: 10 in]
            n108 = call "Sort Array by Column.vi"("Unsorted Array"=w235) -> ("Sorted Array"=w236:string[][])  [unwired: 10 in]
            n109 = call "Sort Array by Column.vi"("Unsorted Array"=w234) -> ("Sorted Array"=w233:string[][])  [unwired: 10 in]
            n110 = property class="MCListbox (strict)"(reference=w245, error in=w242, "ItemNames"=w244) -> (error out=w238:errorcluster)  [unwired: 1 out]
            n111 = Bundle By Name(cluster=w240, "Complete Log"=w236, "Complete Log (Alias)"=w233) -> (w237:refnum<class "Message Log.lvclass">)
          }
          frame "EHL Resize - Value Change" {
            # "Adjusts the width of the columns to the size of the text within the cells"
            n112 = Variant To Data(error in=w257, type=T32 {"String"=""} ("Data"), Variant=w255) -> (data=w254:T32, error out=w251:errorcluster)
            n113 = Unbundle By Name(w254) -> ()  [unwired: 1 out]
            n114 = Unbundle By Name(w253) -> ("Message Log.Ref"=w252:refnum<vi>)
            n115 = call "Size Column Width to Text.vi"("error in"=w251, "MulticolumnListbox"=w252) -> ("error out"=w250:errorcluster)  [unwired: 9 in]
          }
          frame "EHL Filter - Value Change" {
            # "Filter Button has been pressed. Add Element to Filter Data and update the Message Log with the filtered data"
            n116 = call "EHL Filter - Value Change MHLC.vi"("error in (no error)"=w261, "Message Log in"=w259) -> ("error out"=w260:errorcluster, "Message Log out"=w258:refnum<class "Message Log.lvclass">)  [unwired: 8 in]
          }
          frame "EHL Undo Filter - Value Change" {
            # "Remove last applied filter"
            n117 = Variant To Data(error in=w269, type=T33 {"String"=""} ("Data"), Variant=w266) -> (data=w265:T33, error out=w268:errorcluster)
            n118 = Unbundle By Name(w265) -> ()  [unwired: 1 out]
            n119 = call "EHL Undo Filter - Value Change MHLC.vi"("error in (no error)"=w268, "Message Log in"=w263) -> ("error out"=w264:errorcluster, "Message Log out"=w262:refnum<class "Message Log.lvclass">)  [unwired: 8 in]
          }
          frame "EHL Clear Filter - Value Change" {
            # "Scroll to Top"
            # "Delete all elements in the filter element cluster, and call <UI Message Log>"
            n120 = Bundle By Name(cluster=w278, "Filter Message Log?"=FALSE, "Filter Data"=T24[] []) -> (w276:refnum<class "Message Log.lvclass">)
            n121 = call "Write to Filter Log.vi"("Message Log in"=w276) -> ("Message Log out"=w275:refnum<class "Message Log.lvclass">)  [unwired: 9 in, 1 out]
            n122 = call "rql_Update UI Message Log.vi"("error in"=w280, "Message Log in"=w275) -> ("error out"=w271:errorcluster, "dup Message Log out"=w274:refnum<class "Message Log.lvclass">)  [unwired: 8 in]
            n123 = Unbundle By Name(w274) -> ("Message Log.Ref"=w272:refnum<vi>)
            n124 = property class="MCListbox (strict)"(reference=w272, error in=w271, "TopLeft"=T12 {"Row"=0, "Column"=0} ("Top Left Visible Cell")) -> (error out=w270:errorcluster)  [unwired: 1 out]
          }
          frame "EHL Show Application Manager" {
            # "Send Response to Caller to show Application Manager's Front Panel"
            n125 = call "rsp_Show Application Manager.vi"("error in"=w284, "Message Log in"=w282) -> ("error out"=w283:errorcluster, "dup Message Log out"=w281:refnum<class "Message Log.lvclass">)  [unwired: 8 in]
          }
          frame "Update Message Log Columns" {
            # "Workers Local API Request Case"
            n126 = Variant To Data(error in=w300, type=T21 {"Boolean"=FALSE} ("Data"), Variant=w297) -> (data=w296:T21, error out=w299:errorcluster)
            n127 = local read "Visible ML Columns"() -> (w293:bool[])
            n128 = Unbundle By Name(w296) -> ("Boolean"=w285:bool)
            n129 = call "Message Log Headers.vi"() -> ("Message Log Headers"=w294:string[])  [unwired: 11 in]
            n130 = for {
              tunnel: w294 -> [w311]
              shift-right: [w308] -> w291
              shift-left: string[] [] -> [w309]
              tunnel: w293 -> [w307] mode=indexing
              i -> [w312]
              n131 = Index Array(array=w311, index=w312) -> (element=w310:string)
              n132 = case shown="True" w307 {
                tunnel: w310 -> [_ w314]
                tunnel: w309 -> [w313 w316]
                tunnel: [w313 w315] -> w308
                frame False {
                }
                frame True {
                  n133 = Build Array (concatenate)(w316, w314) -> (w315:string[])
                }
              }
            }
            n134 = Unbundle By Name(w289) -> ("Message Log.Ref"=w292:refnum<vi>)
            n135 = property class="MCListbox (strict)"(reference=w292, "ColHdrString"=w291) -> ()  [unwired: 1 in, 2 out]
            n136 = call "rql_Update UI Message Log.vi"("error in"=w299, "Message Log in"=w289) -> ("error out"=w290:errorcluster, "dup Message Log out"=w287:refnum<class "Message Log.lvclass">)  [unwired: 8 in]
            n137 = case shown="True" w285 {
              tunnel: w290 -> [w302 w306]
              tunnel: [w302 w305] -> w288
              tunnel: w287 -> [w301 w304]
              tunnel: [w301 w303] -> w286
              frame False {
              }
              frame True {
                n138 = call "rql_EHL Resize - Value Change.vi"("error in"=w306, "Message Log in"=w304) -> ("error out"=w305:errorcluster, "dup Message Log out"=w303:refnum<class "Message Log.lvclass">)  [unwired: 8 in]
              }
            }
          }
          frame "EHL Logging - Value Change" {
            # "Create Log File if it has not yet been created"
            n139 = Variant To Data(error in=w326, type=T34 {"Boolean"=FALSE} ("Data"), Variant=w322) -> (data=w321:T34, error out=w324:errorcluster)
            n140 = Unbundle By Name(w321) -> ("Boolean"=w320:bool)
            n141 = Bundle By Name(cluster=w325, "Logging?"=w320) -> (w318:refnum<class "Message Log.lvclass">)
            n142 = call "Create Log File.vi"("error in (no error)"=w324, "Message Log in"=w318) -> ("error out"=w319:errorcluster, "Message Log out"=w317:refnum<class "Message Log.lvclass">)  [unwired: 8 in]
          }
          frame "------------- PUBLIC API CASES -------------" {
            # "Start of Workers Public API Cases"
          }
          frame "Show Front Panel" {
            # "Show the front panel of this Worker's Main VI"
            n143 = Variant To Data(error in=w334, type=T35 {"String"=""} ("Data"), Variant=w330) -> (data=w329:T35, error out=w332:errorcluster)
            n144 = Unbundle By Name(w329) -> ()  [unwired: 1 out]
            n145 = invoke class="VI" method="FP.Open"() -> ()  [unwired: 5 in, 5 out]
          }
          frame "Get Shutdown Data" {
            # "Collect the shutdown data from this Worker and send to Caller"
            n146 = control-ref of="Splitter"() -> (w338:refnum<vi>)
            n147 = call "Get Shutdown Data.vi"("error in (no error)"=w341, "Splitter"=w338, "Message Log in"=w336) -> ("error out"=w343:errorcluster, "Data"=w337:T18, "Message Log out"=w335:refnum<class "Message Log.lvclass">)  [unwired: 6 in]
            n148 = Bundle By Name(cluster=T36 {"Config Data"={"Max Num Rows"=0, "Visible Columns"=[], "Splitter Position"=0, "Column Widths"=[], "WinBounds"={"Left"=0, "Top"=0, "Right"=0, "Bottom"=0}, "FP.State"=enum."Invalid", "Monitor"=0, "Logging"=FALSE, "LogBaseFolder"=path ""}} ("Reply Data"), "Config Data"=w337) -> (w344:T36)
            n149 = call-dynamic "Callback Easy Reply.vi"("error in"=w343, "Data"=w344, "Worker"=w335) -> ("error out"=w340:errorcluster, "dup Worker out"=w339:refnum<class "Message Log.lvclass">)  [unwired: 7 in]
          }
          frame "Filter as Enque Worker" {
            # "First, set to String Only"
            # "Enque Worker Actual Column"
            # "Apply filter to Enque Worker column with selected Worker"
            n150 = Variant To Data(error in=w361, type=T37 {"Worker ID"=""} ("Data"), Variant=w358) -> (data=w357:T37, error out=w360:errorcluster)
            n151 = Unbundle By Name(w354) -> ("Filter Type.Ref"=w348:refnum<vi>, "WID Pressed?"=w353:bool)
            n152 = Unbundle By Name(w357) -> ("Worker ID"=w352:string)
            n153 = call <vilib>:"WID to Alias.vi"("WID"=w352) -> ("Alias"=w351:string)
            n154 = Select(t=w352, s=w353, f=w351) -> (s? t:f=w349:string)
            n155 = property class="Enum (strict)"(reference=w348, "Value"=enum16{"string only", "match pattern"}."string only") -> (error out=w345:errorcluster)  [unwired: 1 in, 1 out]
            n156 = Merge Errors(w360, w345) -> (w346:errorcluster)
            n157 = call "Filter String.vi"("error in (no error)"=w346, "Actual Column"=2 ("Column"), "Filter String"=w349, "Message Log in"=w354) -> ("error out"=w356:errorcluster, "Message Log out"=w355:refnum<class "Message Log.lvclass">)  [unwired: 6 in]
          }
          frame "Filter as Deque Worker" {
            # "First, set to String Only"
            # "Enque Worker Actual Column"
            # "Apply filter to Deque Worker column with selected Worker"
            n158 = Variant To Data(error in=w378, type=T38 {"Worker ID"=""} ("Data"), Variant=w375) -> (data=w374:T38, error out=w377:errorcluster)
            n159 = Unbundle By Name(w371) -> ("Filter Type.Ref"=w365:refnum<vi>, "WID Pressed?"=w370:bool)
            n160 = Unbundle By Name(w374) -> ("Worker ID"=w369:string)
            n161 = call <vilib>:"WID to Alias.vi"("WID"=w369) -> ("Alias"=w368:string)
            n162 = Select(t=w369, s=w370, f=w368) -> (s? t:f=w366:string)
            n163 = property class="Enum (strict)"(reference=w365, "Value"=enum16{"string only", "match pattern"}."string only") -> (error out=w362:errorcluster)  [unwired: 1 in, 1 out]
            n164 = Merge Errors(w377, w362) -> (w363:errorcluster)
            n165 = call "Filter String.vi"("error in (no error)"=w363, "Actual Column"=4 ("Column"), "Filter String"=w366, "Message Log in"=w371) -> ("error out"=w373:errorcluster, "Message Log out"=w372:refnum<class "Message Log.lvclass">)  [unwired: 6 in]
          }
          frame "----------- DEBUG CLIENT CASES ------------" {
            # "These cases are called externally by the Debug Client application\nMessages are forwarded to these cases directly by the DS TCP Read Worker"
          }
          frame "Receive New Message" {
            # "This case is called externally by a Worker's Debug Client.\nUpdate the Message Log with the new data"
            n166 = call "Receive and Sort new Message.vi"("error in"=w386, "Data"=w387, "Message Log in"=w388) -> ("error out"=w385:errorcluster, "Message Log out"=w382:refnum<class "Message Log.lvclass">)  [unwired: 7 in]
            n167 = Unbundle By Name(w382) -> ("Paused Pressed?"=w381:bool)
            n168 = case shown="False" w381 {
              tunnel: w385 -> [w392 w393]
              tunnel: [w391 w393] -> w384
              tunnel: w382 -> [w390 w394]
              tunnel: [w389 w394] -> w383
              frame False {
                # "Update immediately\nfor smooth updating"
                n169 = call "rql_Update UI Message Log.vi"("error in"=w392, "Message Log in"=w390) -> ("error out"=w391:errorcluster, "dup Message Log out"=w389:refnum<class "Message Log.lvclass">)  [unwired: 8 in]
              }
              frame True {
              }
            }
          }
        }
        n170 = call-dynamic "Error Handler.vi"("Worker"=w59, "error_in"=w61) -> ("error out"=w64:errorcluster, "Stop Loop"=w57:bool, "Worker out"=w63:refnum<class "Message Log.lvclass">)  [unwired: 7 in]
      }
      n171 = call-dynamic "Setup EHL.vi"("Worker"=w49) -> ("Worker out"=w50:refnum<class "Message Log.lvclass">)  [unwired: 14 in]
      n172 = while "Event Handling Loop" {
        shift-right: [w404] -> w53
        shift-left: w54 -> [w403]
        tunnel: [w399] -> w51
        tunnel: errorcluster {"status"=FALSE, "code"=0, "source"=""} ("error constant") -> [w401]
        shift-right: [w397] -> _
        shift-left: w50 -> [w402]
        stop <- w396 stop-if-true
        # "Event Handling Loop"
        n173 = event shown="[9] \"WID\": Value Change" {
          selector: w403 -> [_ _ _ _ _ _ _ _ _ _ _ _ _ _ _ _ _ _]
          dyn-events: [_ _ _ _ _ _ _ _ _ _ _ _ _ _ _ _ _ _] -> w404
          timeout: 100 -> [_ _ _ _ _ _ _ _ _ _ _ _ _ _ _ _ _ _]
          tunnel: [w409 w413 w418 w425 w432 w468 w475 w479 w486 w493 w497 w501 w505 w509 w512 w523 w530 w536] -> w400
          tunnel: w401 -> [w410 w414 w419 w424 w431 w469 w476 w480 w487 w494 w498 w502 w506 w510 w515 w524 w531 w537]
          tunnel: w402 -> [w408 w412 w417 w423 w430 w466 w474 w478 w485 w492 w496 w500 w504 w508 w517 w522 w529 w535]
          tunnel: [w407 w411 w416 w422 w429 w467 w473 w477 w484 w491 w495 w499 w503 w507 w517 w521 w528 w534] -> w398
          event Timeout {
            n174 = event-data() -> ()  [unwired: 1 in, 1 out]
            n175 = control-ref of="This VI"() -> (w406:refnum<vi>)
            n176 = call "EHL Timeout EHLC.vi"("error in"=w410, "This VI"=w406, "Message Log in"=w408) -> ("error out"=w409:errorcluster, "# elements in queue"=w405:i32, "Message Log out"=w407:refnum<class "Message Log.lvclass">)  [unwired: 6 in]
            n177 = local write "Warning : Message Backlog"(w405) -> ()
          }
          event Value Change {
            n178 = event-data() -> ()  [unwired: 1 in, 1 out]
            n179 = call "rql_EHL Show Application Manager.vi"("error in"=w414, "Message Log in"=w412) -> ("error out"=w413:errorcluster, "dup Message Log out"=w411:refnum<class "Message Log.lvclass">)  [unwired: 8 in]
          }
          event User Event {
            # "This case and its contents must always be included in every EHL that you use, so that the framework can automatically stop the EHL."
            # "EHL Stop Event. This EHL exits from this case."
            n180 = event-data() -> ("Stop Event Data"=w415:variant)  [unwired: 1 in]
            n181 = call-dynamic "EHL Stop - EHL Case.vi"("error in"=w419, "Stop Event Data"=w415, "Worker"=w417) -> ("error out"=w418:errorcluster, "Worker out"=w416:refnum<class "Message Log.lvclass">)  [unwired: 7 in]
          }
          event Panel Close? {
            # "Use this VI when you want to exit this Worker. This VI will call the Start Exiting case of this Worker. This is the correct way to exit your Worker."
            # "Calls the Start Exiting case of this Worker. This will start the exiting sequence of this Worker."
            n182 = event-data() -> ()  [unwired: 1 in, 1 out]
            n183 = call <vilib>:"Read Queue.vi"("Worker_"=w423) -> ("Message Queue out"=w420:refnum<class "Message Queue.lvclass">, "dup Worker_out"=w421:refnum<class "Message Log.lvclass">)  [unwired: 9 in]
            n184 = call-dynamic "Worker Start Exiting.vi"("error_in"=w424, "Message Queue"=w420, "Worker"=w421) -> ("error out"=w425:errorcluster, "dup Worker out"=w422:refnum<class "Message Log.lvclass">)  [unwired: 7 in]
            n185 = event-data("Discard?"=TRUE) -> ()  [unwired: 1 in, 1 out]
          }
          event Menu Selection (User) {
            n186 = event-data() -> ("ItemTag"=w428:string, "MenuRef"=w427:refnum<k9>)  [unwired: 1 in]
            n187 = case shown="\"Online Help\"" w428 {
              selector: w428 -> [_ _ _ w450 _]
              tunnel: [w433 w436 w442 w454 w463] -> w432
              tunnel: w431 -> [w433 w436 w441 w458 w463]
              tunnel: w430 -> [w434 w435 w440 w444 w462]
              tunnel: [w434 w435 w439 w453 w462] -> w429
              tunnel: w427 -> [_ _ _ w457 _]
              frame Default {
              }
              frame "About" {
                n188 = call "About Dialog.vi"() -> ()  [unwired: 12 in]
              }
              frame "Exit" {
                n189 = call <vilib>:"Read Queue.vi"("Worker_"=w440) -> ("Message Queue out"=w437:refnum<class "Message Queue.lvclass">, "dup Worker_out"=w438:refnum<class "Message Log.lvclass">)  [unwired: 9 in]
                n190 = call-dynamic "Worker Start Exiting.vi"("error_in"=w441, "Message Queue"=w437, "Worker"=w438) -> ("error out"=w442:errorcluster, "dup Worker out"=w439:refnum<class "Message Log.lvclass">)  [unwired: 7 in]
              }
              frame "Deque Case", "Deque Worker", "Enque Case", "Enque Worker", "Message", "Priority", "Time/Date" {
                # "Toggle Check mark"
                n191 = call "Message Log Headers.vi"() -> ("Message Log Headers"=w449:string[])  [unwired: 11 in]
                n192 = Get Menu Item Info(7:w450, 8:w458, 11:w457) -> (0:w459:errorcluster, 3:w456:refnum<k9>, 4:w460:bool)  [unwired: 4 out]
                n193 = Not(x=w460) -> (.not. x?=w447:bool)
                n194 = Set Menu Item Info(6:w447, 7:w450, 8:w459, 11:w456) -> (0:w455:errorcluster)  [unwired: 3 in, 1 out]
                n195 = local read "Visible ML Columns"() -> (w452:bool[])
                n196 = Search 1D Array(1D array=w449, element=w450) -> (index of element=w448:i32)  [unwired: 1 in]
                n197 = Replace Array Subset(array=w452, new element=w447, index=w448) -> (w451:bool[])
                n198 = local write "Visible ML Columns"(w451) -> ()
                n199 = call "rql_EHL Clear Filter - Value Change.vi"("error in"=w455, "Message Log in"=w444) -> ("error out"=w445:errorcluster, "dup Message Log out"=w443:refnum<class "Message Log.lvclass">)  [unwired: 8 in]
                n200 = call "rql_Update Message Log Columns.vi"("error in"=w445, "Data in"=T21 {"Boolean"=TRUE}, "Message Log in"=w443) -> ("error out"=w454:errorcluster, "dup Message Log out"=w453:refnum<class "Message Log.lvclass">)  [unwired: 7 in]
              }
              frame "Online Help" {
                n201 = call-poly <vilib>:"Open URL in Default Browser.vi"("URL"="https://workersforlabview.gitbook.io/documentation/v/5.0/workers-tools/workers-tools-menu/workers-debug-server/worker-message-logs") -> ()  [unwired: 5 in, 2 out]
              }
            }
          }
          event Pane Size {
            n202 = event-data() -> ()  [unwired: 1 in, 1 out]
            n203 = control-ref of="Pane"() -> (w465:refnum<vi>)
            n204 = control-ref of="Pane"() -> ()  [unwired: 1 out]
            n205 = control-ref of="Pane 2"() -> (w464:refnum<vi>)
            n206 = call "Scale Front Panel Controls.vi"("error in (no error)"=w469, "Pane 2"=w464, "Pane"=w465, "Message Log in"=w466) -> ("error out"=w468:errorcluster, "Message Log out"=w467:refnum<class "Message Log.lvclass">)  [unwired: 6 in]
          }
          event Value Change {
            n207 = event-data() -> ("NewVal"=w470:T8)  [unwired: 1 in]
            n208 = Bundle By Name(cluster=T34 {"Boolean"=FALSE} ("Data in"), "Boolean"=w470) -> (w471:T34)
            n209 = call "rql_EHL Logging - Value Change.vi"("error in"=w476, "Data in"=w471, "Message Log in"=w474) -> ("error out"=w475:errorcluster, "dup Message Log out"=w473:refnum<class "Message Log.lvclass">)  [unwired: 7 in]
          }
          event Value Change {
            n210 = event-data() -> ()  [unwired: 1 in, 1 out]
            n211 = call "rql_EHL Sort - Value Change.vi"("error in"=w480, "Message Log in"=w478) -> ("error out"=w479:errorcluster, "dup Message Log out"=w477:refnum<class "Message Log.lvclass">)  [unwired: 8 in]
          }
          event Value Change {
            n212 = event-data() -> ("NewVal"=w481:T3)  [unwired: 1 in]
            n213 = Bundle By Name(cluster=T29 {"Boolean"=FALSE} ("Data in"), "Boolean"=w481) -> (w482:T29)
            n214 = call "rql_EHL Pause - Value Change.vi"("error in"=w487, "Data in"=w482, "Message Log in"=w485) -> ("error out"=w486:errorcluster, "dup Message Log out"=w484:refnum<class "Message Log.lvclass">)  [unwired: 7 in]
          }
          event Value Change {
            n215 = event-data() -> ("NewVal"=w488:T2)  [unwired: 1 in]
            n216 = Bundle By Name(cluster=T30 {"Boolean"=FALSE} ("Data in"), "Boolean"=w488) -> (w489:T30)
            n217 = call "rql_EHL WID - Value Change.vi"("error in"=w494, "Data in"=w489, "Message Log in"=w492) -> ("error out"=w493:errorcluster, "dup Message Log out"=w491:refnum<class "Message Log.lvclass">)  [unwired: 7 in]
          }
          event Value Change {
            n218 = event-data() -> ()  [unwired: 1 in, 1 out]
            n219 = call "rql_EHL Resize - Value Change.vi"("error in"=w498, "Message Log in"=w496) -> ("error out"=w497:errorcluster, "dup Message Log out"=w495:refnum<class "Message Log.lvclass">)  [unwired: 8 in]
          }
          event Value Change {
            n220 = event-data() -> ()  [unwired: 1 in, 1 out]
            n221 = call "rql_EHL Filter - Value Change.vi"("error in"=w502, "Message Log in"=w500) -> ("error out"=w501:errorcluster, "dup Message Log out"=w499:refnum<class "Message Log.lvclass">)  [unwired: 8 in]
          }
          event Value Change {
            n222 = event-data() -> ()  [unwired: 1 in, 1 out]
            n223 = call "rql_EHL Undo Filter - Value Change.vi"("error in"=w506, "Message Log in"=w504) -> ("error out"=w505:errorcluster, "dup Message Log out"=w503:refnum<class "Message Log.lvclass">)  [unwired: 8 in]
          }
          event Value Change {
            n224 = event-data() -> ()  [unwired: 1 in, 1 out]
            n225 = call "rql_EHL Clear Filter - Value Change.vi"("error in"=w510, "Message Log in"=w508) -> ("error out"=w509:errorcluster, "dup Message Log out"=w507:refnum<class "Message Log.lvclass">)  [unwired: 8 in]
          }
          event "Message Log": Shortcut Menu Activation? {
            w511 = string[] ["Filter String (Double Click)", "Open Running VI", "Go to Case", "app_separator", "Clear Message Log"] ("item names")
            # "The menu items are hardcoded here\nbecause VIPM loses track of the link\nto the .rtm file (if one is used)"
            n226 = event-data() -> ("MenuRef"=w516:refnum<k9>)  [unwired: 1 in]
            n227 = Delete Menu Items(6:w515, 9:w516) -> (0:w514:errorcluster, 3:w513:refnum<k9>)  [unwired: 2 in]
            n228 = Insert Menu Items(6:w514, 7:w511, 8:w511, 9:w513) -> (0:w512:errorcluster)  [unwired: 2 in, 2 out]
            n229 = event-data() -> ()  [unwired: 2 in, 1 out]
          }
          event "Message Log": Shortcut Menu Selection (User) {
            n230 = event-data() -> ("CtlRef"=w520:refnum<vi>, "Coords"=w519:T39, "ItemPath"=w518:string)  [unwired: 1 in]
            n231 = call "Message Log Shortcut Menu Selection.vi"("ItemPath"=w518, "error in (no error)"=w524, "Coords"=w519, "CtlRef"=w520, "Message Log in"=w522) -> ("error out"=w523:errorcluster, "Message Log out"=w521:refnum<class "Message Log.lvclass">)  [unwired: 5 in]
          }
          event "Message Log": Double Click {
            n232 = event-data() -> ("CtlRef"=w527:refnum<vi>, "Coords"=w526:T39)  [unwired: 1 in]
            n233 = call "Message Log Shortcut Menu Selection.vi"("ItemPath"="Filter String (Double Click)", "error in (no error)"=w531, "Coords"=w526, "CtlRef"=w527, "Message Log in"=w529) -> ("error out"=w530:errorcluster, "Message Log out"=w528:refnum<class "Message Log.lvclass">)  [unwired: 5 in]
          }
          event "Message Log": Mouse Down {
            n234 = event-data() -> ("CtlRef"=w533:refnum<vi>, "Coords"=w532:T39)  [unwired: 1 in]
            n235 = call "Message Log Mouse Down EHLC.vi"("error in (no error)"=w537, "Coords"=w532, "CtlRef"=w533, "Message Log in"=w535) -> ("error out"=w536:errorcluster, "Message Log out"=w534:refnum<class "Message Log.lvclass">)  [unwired: 6 in]
          }
        }
        n236 = call-dynamic "Error Handler.vi"("Worker"=w398, "error_in"=w400) -> ("error out"=w399:errorcluster, "Stop Loop"=w396:bool, "Worker out"=w397:refnum<class "Message Log.lvclass">)  [unwired: 7 in]
      }
    }
    frame Error {
      n237 = call-dynamic "Error Handler.vi"("Worker"=w539, "error_in"=w542) -> ("error out"=w540:errorcluster, "Worker out"=w538:refnum<class "Message Log.lvclass">)  [unwired: 7 in, 1 out]
    }
  }
  n238 = Unregister For Events(event registration refnum=w21, error in=w22) -> (error out=w23:errorcluster)
  n239 = Merge Errors(w23, w16) -> (w20:errorcluster)
  n240 = call-dynamic "Exited Notify and Cleanup.vi"("error_in"=w20, "Worker"=w19) -> ("error out"=→"error out":errorcluster, "dup Worker out"=→"Message Log out":refnum<class "Message Log.lvclass">)  [unwired: 8 in]
